vi "Get Plugin UIPs.vi"() -> (2 "UIPs":refnum<class "UIP Interface.lvclass">[](array[class]))   [LabVIEW 2020, in "UIM.lvlib" / "UIM.lvclass"]
doc: "Returns a list of all UIPs loaded from the <b><user data>\\LabVIEW Data\\UIP</b> folder. You can place UIPs in that folder if you want them to be loaded dynamically by LabVIEW.\n\n<b>NOTE</b> This method is invoked each time UIM is obtained. This means that Quick Drop and Right Click menu options will also use these dynamic plugin UIPs."
uses:
  UIM.lvclass
  UIP Interface/UIP Interface.lvclass
  <vilib>/Utility/sysdir.llb/System Directory Type.ctl
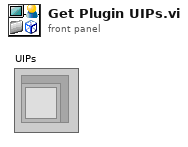
[diagram p1: front panel]
types:
  T1 = typedef "System Directory Type.ctl" = i32
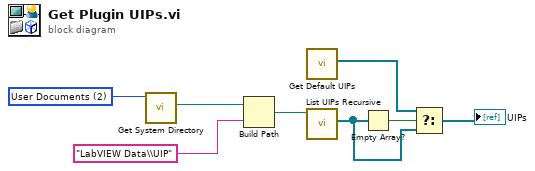
[diagram p0: block diagram]
diagram:
  w8 = T1 2 items=["User Home"=0, "User Desktop"=1, "User Documents"=2, "User Application Data"=3, "User Preferences"=4, "User Temporary"=5, "Public Documents"=6, "Public Application Data"=7, "Public Preferences"=8, "Public Cache"=13, "System Core Libraries"=9, "System Installed Libraries"=10, "Application Files"=11, "Boot Volume Root"=12] ("system directory type")
  n1 = call <vilib>:"Get System Directory.vi"("system directory type"=w8) -> ("system directory"=w7:path)  [unwired: 10 in]
  n2 = Build Path(base path=w7, name or relative path="LabVIEW Data\\UIP") -> (appended path=w5:path)
  n3 = call "Get Default UIPs.vi"() -> ("UIPs"=w3:refnum<class "UIP Interface.lvclass">[])  [unwired: 11 in]
  n4 = call "List UIPs Recursive.vi"("Plugin Folder Path"=w5) -> ("UIPs"=w2:refnum<class "UIP Interface.lvclass">[])  [unwired: 9 in, 1 out]
  n5 = Empty Array?(array=w2) -> (empty?=w4:bool)
  n6 = Select(t=w3, s=w4, f=w2) -> (s? t:f=→"UIPs":refnum<class "UIP Interface.lvclass">[])
